vi "Set Delay.vi"(8 "error in":errorcluster, 9 "Line":i32, 10 "PWM Delay":dbl format="%.3g", 11 "BNT_ULx-MCSV-DOPWM in":refnum<class "BNT_ULx-MCSV-DOPWM.lvclass">) -> (0 "error out":errorcluster, 3 "BNT_ULx-MCSV-DOPWM out":refnum<class "BNT_ULx-MCSV-DOPWM.lvclass">)   [LabVIEW 2020, in "BNT_ULx.lvlib" / "BNT_ULx-MCSV-DOPWM.lvclass"]
doc: "Set pulse delay at index."
uses:
  BNT_ULx-MCSV-DOPWM.lvclass
  BNT_ULx-MCSV-DOPWM.lvclass/BNT_ULx-MCSV-DOPWM.ctl
  CSPP_Core/Classes/CSPP_ProcessVariables/PVConnection/PVConnection.lvclass
  CSPP_Core/Classes/CSPP_ProcessVariables/ProcessVariable/PV.lvclass
  BNT_ULx-MCSV/BNT_ULx-MCSV.lvclass
  C:/User/Brand/LVP/CSPP/CSPP-Template/Packages/BNT_ULx/BNT_ULx-MCSV/BNT_ULx-MCSV/BNT_ULx-MCSV.lvclass
  C:/User/Brand/LVP/CSPP/CSPP-Template/Packages/CSPP_Core/Actors/CSPP_DeviceActor/CSPP_DeviceActor.lvclass
  C:/User/Brand/LVP/CSPP/CSPP-Template/Packages/CSPP_Core/Actors/CSPP_BaseActor/CSPP_BaseActor.lvclass
  C:/Program Files (x86)/National Instruments/LabVIEW 2020/vi.lib/ActorFramework/Actor/Actor.lvclass
  C:/User/Brand/LVP/CSPP/CSPP-Template/Packages/BNT_ULx/BNT_ULx-MCSV/BNT_ULx-MCSV-DOPWM/BNT_ULx-MCSV-DOPWM.lvclass
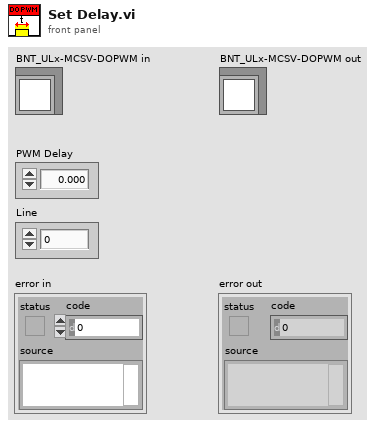
[diagram p1: front panel]
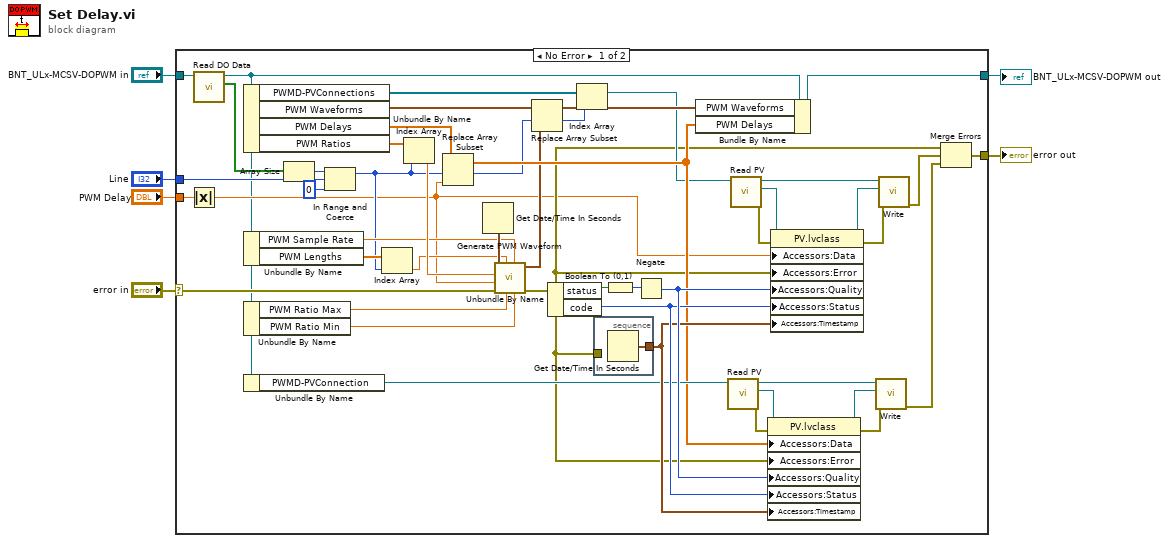
[diagram p0: block diagram]
diagram:
  n1 = case shown="No Error" "error in" {
    selector: "error in" -> [w22 w55]
    tunnel: [w49 w55] -> w2
    tunnel: [w47 w54] -> w1
    tunnel: "BNT_ULx-MCSV-DOPWM in" -> [w8 w54]
    tunnel: "PWM Delay" -> [w14 _]
    tunnel: "Line" -> [w24 _]
    frame No Error {
      n2 = Absolute Value(x=w14) -> (abs(x)=w10:dbl)
      n3 = call "Read DO Data.vi"("BNT_DAQmx-MCSV in"=w8) -> ("DO Data"=w9:bool[], "BNT_DAQmx-MCSV out"=w7:refnum<class "BNT_ULx-MCSV-DOPWM.lvclass">)  [unwired: 8 in, 1 out]
      n4 = Unbundle By Name(w7) -> ("PWMD-PVConnections"=w48:refnum<class "PVConnection.lvclass">[], "PWM Waveforms"=w35:waveform(dbl)[], "PWM Delays"=w36:dbl[], "PWM Ratios"=w23:dbl[])
      n5 = Unbundle By Name(w7) -> ("PWM Sample Rate"=w15:dbl[unit], "PWM Lengths"=w13:dbl[unit][])
      n6 = Unbundle By Name(w7) -> ("PWM Ratio Max"=w17:dbl, "PWM Ratio Min"=w16:dbl)
      n7 = Unbundle By Name(w7) -> ("PWMD-PVConnection"=w37:refnum<class "PVConnection.lvclass">)
      n8 = Array Size(array=w9) -> (size(s)=w26:i32)
      n9 = In Range and Coerce(upper limit=w26, x=w24, lower limit=0) -> (coerced(x)=w11:i32)  [unwired: 1 out]
      n10 = Index Array(array=w13, index=w11) -> (element=w12:dbl[unit])
      n11 = Index Array(array=w23, index=w11) -> (element=w18:dbl)
      n12 = Replace Array Subset(array=w36, new element=w10, index=w11) -> (w33:dbl[])
      n13 = Get Date/Time In Seconds() -> (seconds since 1Jan1904=w20:timestamp)
      n14 = call "Generate PWM Waveform.vi"("PWM Ratio Min"=w16, "PWM Sample Rate"=w15, "PWM Ratio Max"=w17, "PWM Length"=w12, "error in (no error)"=w22, "PWM Delay"=w10, "PWM Ratio"=w18, "Timestamp"=w20) -> ("error out"=w19:errorcluster, "PWM Waveform"=w21:waveform(dbl))  [unwired: 2 in]
      n15 = Replace Array Subset(array=w35, new element=w21, index=w11) -> (w34:waveform(dbl)[])
      n16 = Unbundle By Name(w19) -> ("status"=w51:bool, "code"=w40:i32)
      n17 = Index Array(array=w48, index=w11) -> (element=w32:refnum<class "PVConnection.lvclass">)
      n18 = stacked-sequence {
        tunnel: [w53] -> w39
        tunnel: w19 -> [_]
        frame #0 {
          n19 = Get Date/Time In Seconds() -> (seconds since 1Jan1904=w53:timestamp)
        }
      }
      n20 = Boolean To (0,1)(Boolean=w51) -> (0, 1=w52:i16)
      n21 = Negate(x=w52) -> (-x=w41:i16)
      n22 = Bundle By Name(cluster=w7, "PWM Waveforms"=w34, "PWM Delays"=w33) -> (w47:refnum<class "BNT_ULx-MCSV-DOPWM.lvclass">)
      n23 = call "Read PV.vi"("PVConnection in"=w37) -> ("error out"=w46:errorcluster, "PV"=w45:refnum<class "PV.lvclass">, "PVConnection out"=w44:refnum<class "PVConnection.lvclass">)  [unwired: 8 in]
      n24 = call "Read PV.vi"("PVConnection in"=w32) -> ("error out"=w27:errorcluster, "PV"=w28:refnum<class "PV.lvclass">, "PVConnection out"=w29:refnum<class "PVConnection.lvclass">)  [unwired: 8 in]
      n25 = property class="PV.lvclass"(reference=w45, error in=w46, "Accessors:Data"=w33, "Accessors:Error"=w19, "Accessors:Quality"=w41, "Accessors:Status"=w40, "Accessors:Timestamp"=w39) -> (reference out=w42:refnum<class "PV.lvclass">, error out=w43:errorcluster)
      n26 = property class="PV.lvclass"(reference=w28, error in=w27, "Accessors:Data"=w10, "Accessors:Error"=w19, "Accessors:Quality"=w41, "Accessors:Status"=w40, "Accessors:Timestamp"=w39) -> (reference out=w31:refnum<class "PV.lvclass">, error out=w30:errorcluster)
      n27 = call "Write.vi"("error in (no error)"=w43, "PV"=w42, "PVConnection in"=w44) -> ("error out"=w38:errorcluster)  [unwired: 6 in, 2 out]
      n28 = call "Write.vi"("error in (no error)"=w30, "PV"=w31, "PVConnection in"=w29) -> ("error out"=w50:errorcluster)  [unwired: 6 in, 2 out]
      n29 = Merge Errors(w19, w50, w38) -> (w49:errorcluster)
    }
    frame Error {
    }
  }
  "error out" <- w2
  "BNT_ULx-MCSV-DOPWM out" <- w1
